vi "PCX-7420.vi"() -> ()   [LabVIEW 2012]
uses:
  <vilib>/Instr/_visa.llb/VISA Configure Serial Port (Instr).vi
panel:
  in  "power on exit":bool
  in  "FORCE EXIT":bool
  out "Output Warning":bool
  in  "PCX-740":enum32{"Control and Status"}(tab)
  in  "Amp On/Off":bool
  in  "INT TRIG FREQ":i32=7000 min=1000 max=100000 step=1000
  in  "MAIN PULSEWIDTH msec":dbl=1.0 min=0.05 max=5000.0 step=0.001 format="%.3g"
  in  "BIAS PULSEWIDTH msec":dbl=0.025 min=0.0 max=25000.0 step=0.001 format="%.3f"
  in  "BIAS CURRENT (A)":dbl min=0.0 max=5.8 step=0.001 format="%.3f"
  in  "MAIN CURRENT (A)":dbl=10.0 min=0.0 max=15.7 step=0.001 format="%.3g"
  in  "TRIGGER SOURCE":u16(ring)=1 items=["Internal", "External"]
  in  "EXT TRIG TERM (Ohms)":i32=10000 min=50 max=10000 step=1
  in  "COMM PORT":refnum<visa-resource-name>="PCX7420-RS232"
  out "Int Trig Freq":string="9000 Hz\n"
  out "Main Current":string="10000 mAmps\n"
  out "Main Pulsewidth":string="1100 nsec\n"
  out "Bias Current":string="0 mAmps\n"
  out "Bias Pulsewidth":string="25 nsec\n"
  out "Ext Trig Term":string="10k Ohms\n"
  in  "Enable Output":bool=TRUE
  in  "Set Values":bool
  out "Temp Out (C)":dbl=30.0
  out "Temp In (C)":dbl=27.0
  out "Rear Enable":bool=TRUE
  out "Keyswitch Enable":bool=TRUE
  out "Error Out":errorcluster
  in  "EXIT":bool
  # "PCX\nRESPONSE"
  # "PCX\nCONTROLS"
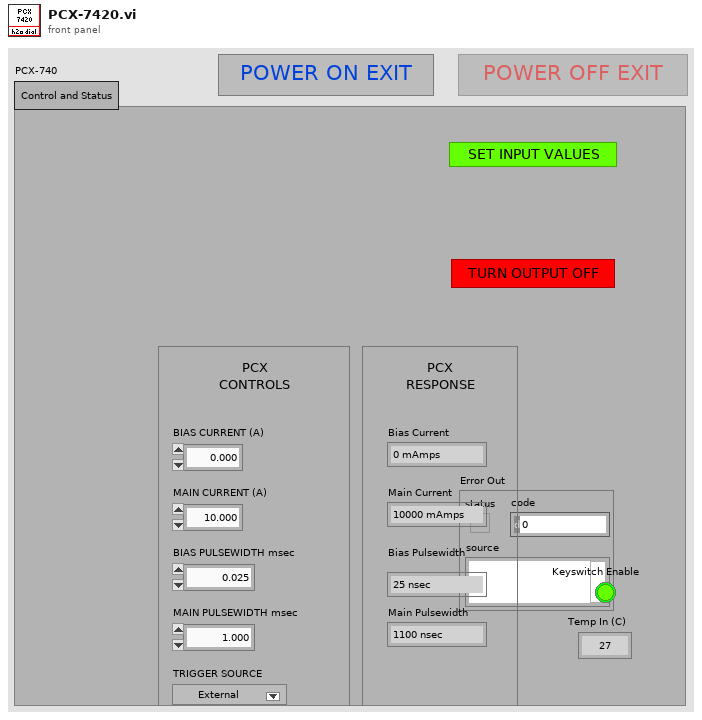
[diagram p1: front panel]
types:
  T1 = enum16{"*IDN?", "BIAS:CURRENT:SETPOINT?", "BIAS:CURRENT:SETPOINT", "FAULT?", "FAULT:CLEAR:ALL", "MAIN:CURRENT:SETPOINT?", "MAIN:CURRENT:SETPOINT", "OUTPUT?", "OUTPUT:DISABLE", "OUTPUT:ENABLE", "*RECALL", "*SAVE", "STATUS:KEYSWITCH?", "STATUS:REAR:ENABLE?", "TEMP:EXHAUST?", "TEMP:IN?", "TRIG?", "TRIG:EXTERNAL", "TRIG:INTERNAL", "TRIG:EXT:TERM?", "TRIG:EXT:TERM", "TRIG:INT:FREQ?", "TRIG:INT:FREQ", "TRIG:INT:BIAS:PULSEWIDTH?", "TRIG:INT:BIAS:PULSEWIDTH", "TRIG:INT:MAIN:PULSEWIDTH?", "TRIG:INT:MAIN:PULSEWIDTH"}
  T2 = enum16{"*IDN?", "BIAS:CURRENT:SETPOINT?", "BIAS:CURRENT:SETPOINT", "FAULT?", "FAULT:CLEAR:ALL", "MAIN:CURRENT:SETPOINT?", "MAIN:CURRENT:SETPOINT", "OUTPUT?", "OUTPUT:DISABLE", "OUTPUT:ENABLE", "*RECALL", "*SAVE", "STATUS:KEYSWITCH?", "STATUS:REAR:ENABLE?", "TEMP:EXHAUST?", "TEMP:IN?", "TRIG?", "TRIG:EXTERNAL", "TRIG:INTERNAL", "TRIG:EXT:TERM?", "TRIG:EXT:TERM", "TRIG:INT:FREQ?", "TRIG:INT:FREQ", "TRIG:INT:BIAS:PULSEWIDTH?", "TRIG:INT:BIAS:PULSEWIDTH", "TRIG:INT:MAIN:PULSEWIDTH?", "TRIG:INT:MAIN:PULSEWIDTH"}[]
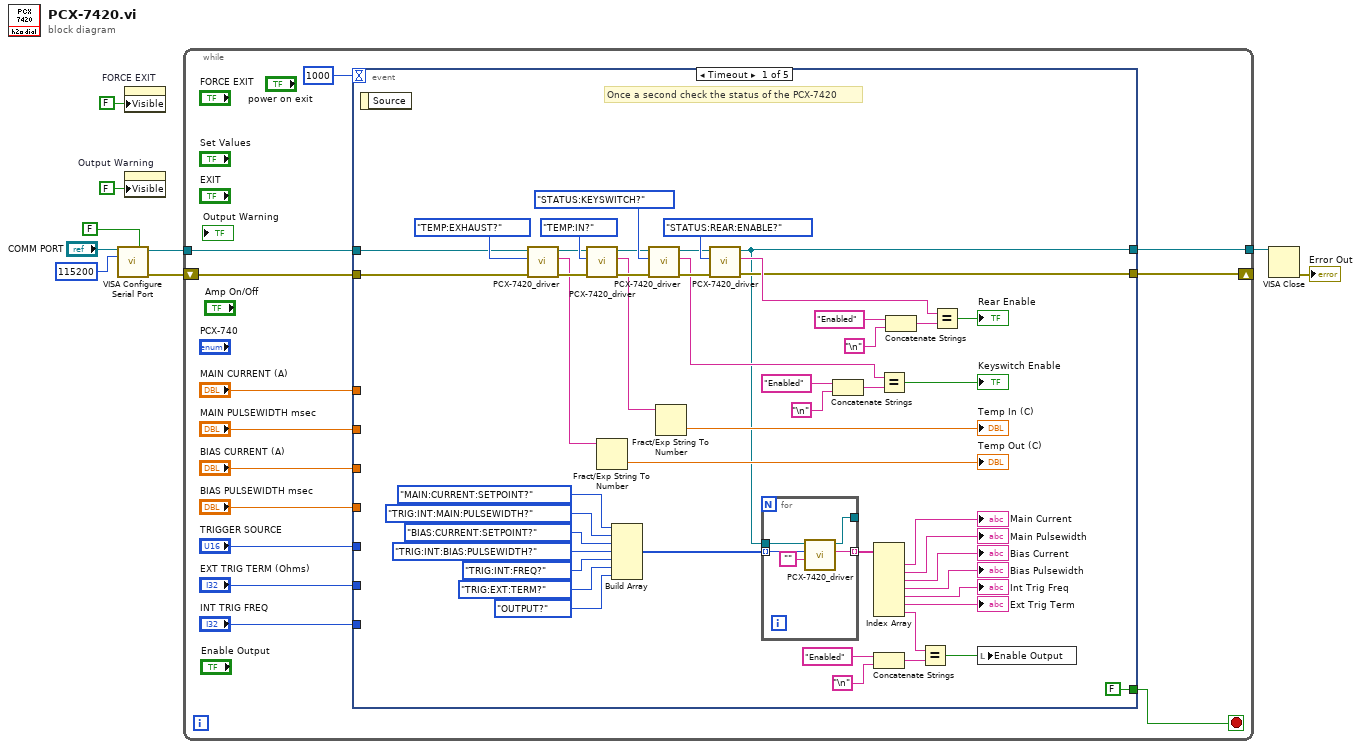
[diagram p0: block diagram]
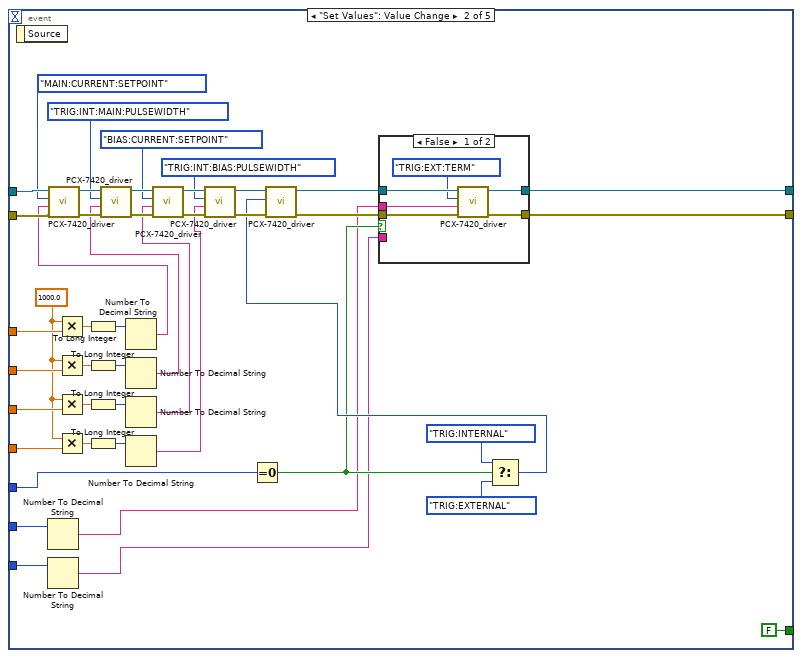
[diagram p2: hidden frame]
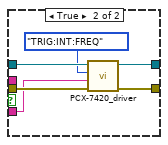
[diagram p3: hidden frame]
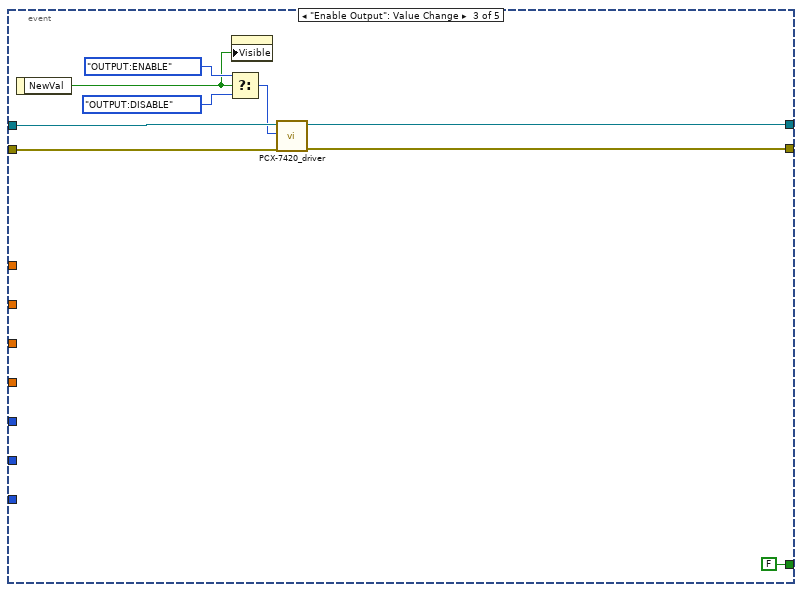
[diagram p4: hidden frame]
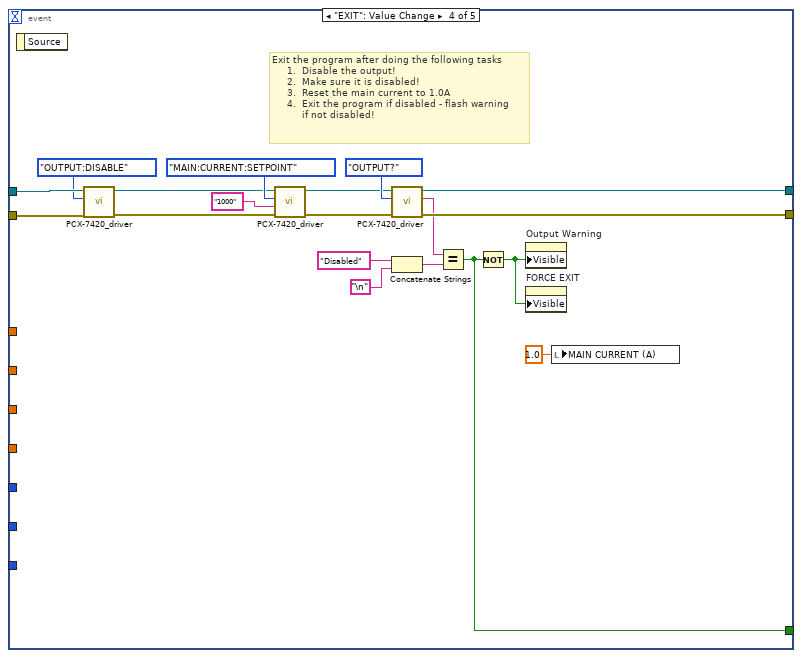
[diagram p5: hidden frame]
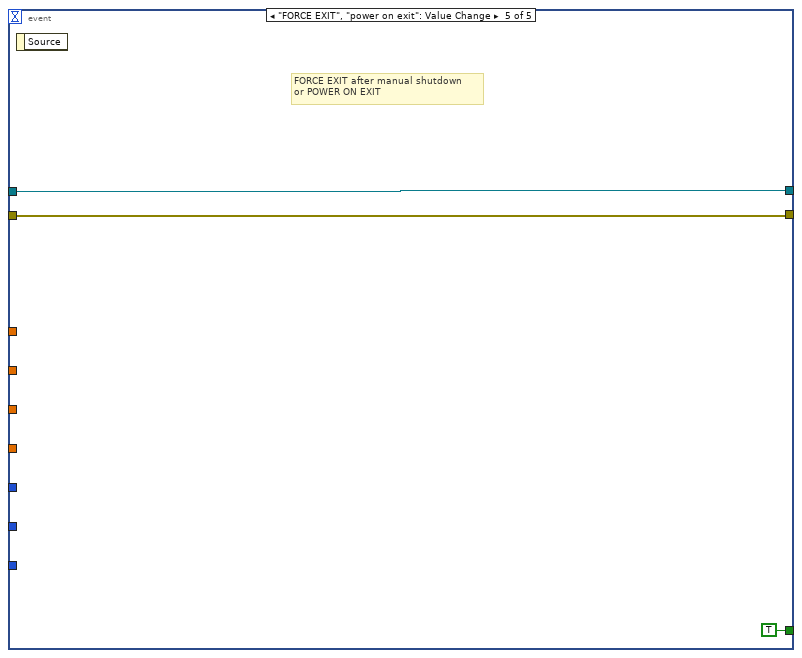
[diagram p6: hidden frame]
diagram:
  n1 = call-poly "VISA Configure Serial Port"("VISA resource name"="COMM PORT", "Enable Termination\nChar (T)"=FALSE ("Enable Termination\nChar (T)"), "baud rate (9600)"=u32 115200) -> ("VISA resource name out"=w5:refnum<visa-resource-name>, "error out"=w4:errorcluster)  [unwired: 11 in]
  n2 = property on="FORCE EXIT" class="Bool"("Visible"=FALSE) -> ()  [unwired: 2 in, 2 out]
  n3 = property on="Output Warning" class="Bool"("Visible"=FALSE) -> ()  [unwired: 2 in, 2 out]
  n4 = while {
    tunnel: w5 -> [w22]
    shift-right: [w20] -> _
    shift-left: w4 -> [w21]
    tunnel: [w19] -> w3
    stop <- w18 stop-if-true
    n5 = event shown="[0] Timeout" {
      selector: _ -> [_ _ _ _ _]
      dyn-events: _ -> [_ _ _ _ _]
      timeout: 1000 -> [_ _ _ _ _]
      tunnel: w22 -> [w41 w121 w141 w161 w163]
      tunnel: w21 -> [w42 w120 w140 w160 w162]
      tunnel: [w29 w81 w137 w159 w163] -> w19
      tunnel: [w30 w80 w138 w158 w162] -> w20
      tunnel: [FALSE FALSE FALSE w150 TRUE] -> w18
      tunnel: "MAIN CURRENT (A)" -> [_ w116 _ _ _]
      tunnel: "MAIN PULSEWIDTH msec" -> [_ w117 _ _ _]
      tunnel: "BIAS CURRENT (A)" -> [_ w118 _ _ _]
      tunnel: "BIAS PULSEWIDTH msec" -> [_ w119 _ _ _]
      tunnel: "TRIGGER SOURCE" -> [_ w91 _ _ _]
      tunnel: "EXT TRIG TERM (Ohms)" -> [_ w106 _ _ _]
      tunnel: "INT TRIG FREQ" -> [_ w79 _ _ _]
      event Timeout {
        # "Once a second check the status of the PCX-7420"
        n6 = event-data() -> ()  [unwired: 1 in, 1 out]
        n7 = call "PCX-7420_driver.vi"("error in"=w42, "PCX-7420 COMMANDS"=T1."TEMP:EXHAUST?", "Comm Port"=w41) -> ("error out"=w65:errorcluster, "read buffer"=w56:string, "Comm Port"=w68:refnum<visa-resource-name>)  [unwired: 6 in]
        n8 = call "PCX-7420_driver.vi"("error in"=w65, "PCX-7420 COMMANDS"=T1."TEMP:IN?", "Comm Port"=w68) -> ("error out"=w64:errorcluster, "read buffer"=w55:string, "Comm Port"=w62:refnum<visa-resource-name>)  [unwired: 6 in]
        n9 = Fract/Exp String To Number(string=w56) -> (number=→"Temp Out (C)":dbl)  [unwired: 3 in, 1 out]
        n10 = Build Array(T1."MAIN:CURRENT:SETPOINT?" ("PCX-7420 COMMANDS"), T1."TRIG:INT:MAIN:PULSEWIDTH?" ("PCX-7420 COMMANDS"), T1."BIAS:CURRENT:SETPOINT?" ("PCX-7420 COMMANDS"), T1."TRIG:INT:BIAS:PULSEWIDTH?" ("PCX-7420 COMMANDS"), T1."TRIG:INT:FREQ?" ("PCX-7420 COMMANDS"), T1."TRIG:EXT:TERM?" ("PCX-7420 COMMANDS"), T1."OUTPUT?" ("PCX-7420 COMMANDS")) -> (w44:T2)
        n11 = call "PCX-7420_driver.vi"("error in"=w64, "PCX-7420 COMMANDS"=T1."STATUS:KEYSWITCH?", "Comm Port"=w62) -> ("error out"=w63:errorcluster, "read buffer"=w53:string, "Comm Port"=w61:refnum<visa-resource-name>)  [unwired: 6 in]
        n12 = Fract/Exp String To Number(string=w55) -> (number=→"Temp In (C)":dbl)  [unwired: 3 in, 1 out]
        n13 = call "PCX-7420_driver.vi"("error in"=w63, "PCX-7420 COMMANDS"=T1."STATUS:REAR:ENABLE?", "Comm Port"=w61) -> ("error out"=w30:errorcluster, "read buffer"=w51:string, "Comm Port"=w29:refnum<visa-resource-name>)  [unwired: 6 in]
        n14 = for {
          tunnel: w44 -> [w76] mode=indexing
          tunnel: w29 -> [w75]
          tunnel: [w73] -> w43 mode=indexing
          tunnel: [w72] -> _
          n15 = call "PCX-7420_driver.vi"("INPUT VALUE"="", "PCX-7420 COMMANDS"=w76, "Comm Port"=w75) -> ("read buffer"=w73:string, "Comm Port"=w72:refnum<visa-resource-name>)  [unwired: 6 in, 1 out]
        }
        n16 = Concatenate Strings("Enabled" ("x"), "\n") -> (w54:string)
        n17 = Index Array(array=w43) -> (element #1=→"Main Current":string, element #2=→"Main Pulsewidth":string, element #3=→"Bias Current":string, element #4=→"Bias Pulsewidth":string, element #5=→"Int Trig Freq":string, element #6=→"Ext Trig Term":string, element #7=w24:string)  [unwired: 7 in]
        n18 = Concatenate Strings("Enabled" ("x"), "\n") -> (w25:string)
        n19 = Equal?(x=w53, y=w54) -> (x = y?=→"Keyswitch Enable":bool)
        n20 = Concatenate Strings("Enabled" ("x"), "\n") -> (w52:string)
        n21 = Equal?(x=w24, y=w25) -> (x = y?=w23:bool)
        n22 = Equal?(x=w51, y=w52) -> (x = y?=→"Rear Enable":bool)
        n23 = local write "Enable Output"(w23) -> ()
      }
      event "Set Values": Value Change {
        w115 = 1000.0 ("x")
        n24 = event-data() -> ()  [unwired: 1 in, 1 out]
        n25 = Number To Decimal String(number=w106) -> (decimal integer string=w82:string)  [unwired: 1 in]
        n26 = Number To Decimal String(number=w79) -> (decimal integer string=w78:string)  [unwired: 1 in]
        n27 = Multiply(x=w115, y=w116) -> (x*y=w114:dbl)
        n28 = Multiply(x=w115, y=w117) -> (x*y=w113:dbl)
        n29 = Multiply(x=w115, y=w118) -> (x*y=w112:dbl)
        n30 = Multiply(x=w115, y=w119) -> (x*y=w111:dbl)
        n31 = To Long Integer(number=w114) -> (32bit integer=w107:i32)
        n32 = To Long Integer(number=w113) -> (32bit integer=w108:i32)
        n33 = To Long Integer(number=w112) -> (32bit integer=w109:i32)
        n34 = To Long Integer(number=w111) -> (32bit integer=w110:i32)
        n35 = Number To Decimal String(number=w107) -> (decimal integer string=w104:string)  [unwired: 1 in]
        n36 = call "PCX-7420_driver.vi"("error in"=w120, "INPUT VALUE"=w104, "PCX-7420 COMMANDS"=T1."MAIN:CURRENT:SETPOINT", "Comm Port"=w121) -> ("error out"=w100:errorcluster, "Comm Port"=w103:refnum<visa-resource-name>)  [unwired: 5 in, 1 out]
        n37 = Number To Decimal String(number=w108) -> (decimal integer string=w96:string)  [unwired: 1 in]
        n38 = call "PCX-7420_driver.vi"("error in"=w100, "INPUT VALUE"=w96, "PCX-7420 COMMANDS"=T1."TRIG:INT:MAIN:PULSEWIDTH", "Comm Port"=w103) -> ("error out"=w99:errorcluster, "Comm Port"=w102:refnum<visa-resource-name>)  [unwired: 5 in, 1 out]
        n39 = Number To Decimal String(number=w109) -> (decimal integer string=w94:string)  [unwired: 1 in]
        n40 = Number To Decimal String(number=w110) -> (decimal integer string=w92:string)  [unwired: 1 in]
        n41 = call "PCX-7420_driver.vi"("error in"=w99, "INPUT VALUE"=w94, "PCX-7420 COMMANDS"=T1."BIAS:CURRENT:SETPOINT", "Comm Port"=w102) -> ("error out"=w98:errorcluster, "Comm Port"=w101:refnum<visa-resource-name>)  [unwired: 5 in, 1 out]
        n42 = call "PCX-7420_driver.vi"("error in"=w98, "INPUT VALUE"=w92, "PCX-7420 COMMANDS"=T1."TRIG:INT:BIAS:PULSEWIDTH", "Comm Port"=w101) -> ("error out"=w88:errorcluster, "Comm Port"=w87:refnum<visa-resource-name>)  [unwired: 5 in, 1 out]
        n43 = Equal To 0?(x=w91) -> (x = 0?=w83:bool)
        n44 = Select(t=T1."TRIG:INTERNAL" ("PCX-7420 COMMANDS"), s=w83, f=T1."TRIG:EXTERNAL" ("PCX-7420 COMMANDS")) -> (s? t:f=w86:T1)
        n45 = call "PCX-7420_driver.vi"("error in"=w88, "PCX-7420 COMMANDS"=w86, "Comm Port"=w87) -> ("error out"=w84:errorcluster, "Comm Port"=w85:refnum<visa-resource-name>)  [unwired: 6 in, 1 out]
        n46 = case shown="False" w83 {
          tunnel: w85 -> [w127 w133]
          tunnel: w84 -> [w126 w132]
          tunnel: [w125 w131] -> w81
          tunnel: [w124 w130] -> w80
          tunnel: w82 -> [w123 _]
          tunnel: w78 -> [_ w128]
          frame False {
            n47 = call "PCX-7420_driver.vi"("error in"=w126, "INPUT VALUE"=w123, "PCX-7420 COMMANDS"=T1."TRIG:EXT:TERM", "Comm Port"=w127) -> ("error out"=w124:errorcluster, "Comm Port"=w125:refnum<visa-resource-name>)  [unwired: 5 in, 1 out]
          }
          frame True {
            n48 = call "PCX-7420_driver.vi"("error in"=w132, "INPUT VALUE"=w128, "PCX-7420 COMMANDS"=T1."TRIG:INT:FREQ", "Comm Port"=w133) -> ("error out"=w130:errorcluster, "Comm Port"=w131:refnum<visa-resource-name>)  [unwired: 5 in, 1 out]
          }
        }
      }
      event "Enable Output": Value Change {
        n49 = event-data() -> ("NewVal"=w134:bool)  [unwired: 1 in]
        n50 = Select(t=T1."OUTPUT:ENABLE" ("PCX-7420 COMMANDS"), s=w134, f=T1."OUTPUT:DISABLE" ("PCX-7420 COMMANDS")) -> (s? t:f=w139:T1)
        n51 = property on="Amp On/Off" class="Bool"("Visible"=w134) -> ()  [unwired: 2 in, 2 out]
        n52 = call "PCX-7420_driver.vi"("error in"=w140, "PCX-7420 COMMANDS"=w139, "Comm Port"=w141) -> ("error out"=w138:errorcluster, "Comm Port"=w137:refnum<visa-resource-name>)  [unwired: 6 in, 1 out]
      }
      event "EXIT": Value Change {
        # "Exit the program after doing the following tasks\n     1.  Disable the output!\n     2.  Make sure it is disabled!\n     3.  Reset the main current to 1.0A\n     4.  Exit the program if disabled - flash warning\n          if not disabled!"
        n53 = event-data() -> ()  [unwired: 1 in, 1 out]
        n54 = call "PCX-7420_driver.vi"("error in"=w160, "PCX-7420 COMMANDS"=T1."OUTPUT:DISABLE", "Comm Port"=w161) -> ("error out"=w146:errorcluster, "Comm Port"=w147:refnum<visa-resource-name>)  [unwired: 6 in, 1 out]
        n55 = call "PCX-7420_driver.vi"("error in"=w146, "INPUT VALUE"="1000", "PCX-7420 COMMANDS"=T1."MAIN:CURRENT:SETPOINT", "Comm Port"=w147) -> ("error out"=w144:errorcluster, "Comm Port"=w145:refnum<visa-resource-name>)  [unwired: 5 in, 1 out]
        n56 = call "PCX-7420_driver.vi"("error in"=w144, "PCX-7420 COMMANDS"=T1."OUTPUT?", "Comm Port"=w145) -> ("error out"=w158:errorcluster, "read buffer"=w152:string, "Comm Port"=w159:refnum<visa-resource-name>)  [unwired: 6 in]
        n57 = Concatenate Strings("Disabled" ("x"), "\n") -> (w153:string)
        n58 = Equal?(x=w152, y=w153) -> (x = y?=w150:bool)
        n59 = Not(x=w150) -> (.not. x?=w151:bool)
        n60 = property on="Output Warning" class="Bool"("Visible"=w151) -> ()  [unwired: 2 in, 2 out]
        n61 = property on="FORCE EXIT" class="Bool"("Visible"=w151) -> ()  [unwired: 2 in, 2 out]
        n62 = local write "MAIN CURRENT (A)"(1.0 ("MAIN CURRENT (A)")) -> ()
      }
      event "FORCE EXIT", "power on exit": Value Change {
        # "FORCE EXIT after manual shutdown\nor POWER ON EXIT"
        n63 = event-data() -> ()  [unwired: 1 in, 1 out]
      }
    }
  }
  n64 = VISA Close(VISA resource name=w3) -> (error out=→"Error Out":errorcluster)  [unwired: 1 in]
